vi "Encoder Counter.vi"(2 "Encoder Full Rotations (n-1)":i32, 3 "Encoder Fraction of one Rotation (n-1)":i32, 4 "Counts per Rotation":i32, 5 "Change in Encoder Value":i32) -> (0 "Encoder Full Rotations (n)":i32, 1 "Encoder Fraction of one Rotation (n)":i32)   [LabVIEW 2009]
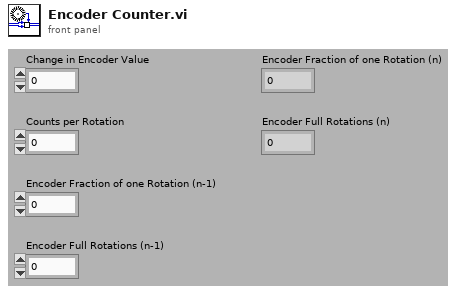
[diagram p1: front panel]
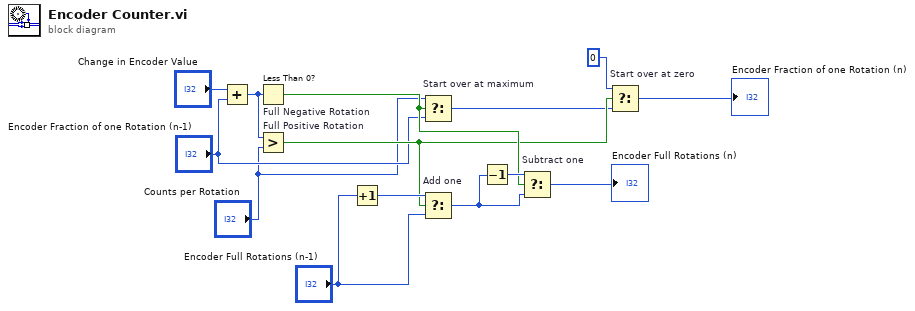
[diagram p0: block diagram]
diagram:
  n1 = Add(x="Change in Encoder Value", y="Encoder Fraction of one Rotation (n-1)") -> (x+y=w1:i32)
  n2 = Less Than 0? "Full Negative Rotation"(x=w1) -> (x < 0?=w8:bool)
  n3 = Greater? "Full Positive Rotation"(x=w1, y="Counts per Rotation") -> (0:w7:bool)
  n4 = Increment(x="Encoder Full Rotations (n-1)") -> (x+1=w9:i32)
  n5 = Select "Start over at maximum"(t="Counts per Rotation", s=w8, f="Encoder Fraction of one Rotation (n-1)") -> (s? t:f=w5:i32)
  n6 = Select "Add one"(t=w9, s=w7, f="Encoder Full Rotations (n-1)") -> (s? t:f=w12:i32)
  n7 = Decrement(x=w12) -> (x-1=w10:i32)
  n8 = Select "Subtract one"(t=w10, s=w8, f=w12) -> (s? t:f=→"Encoder Full Rotations (n)":i32)
  n9 = Select "Start over at zero"(t=0, s=w7, f=w5) -> (s? t:f=→"Encoder Fraction of one Rotation (n)":i32)
